vi "T3AWG Pick Rate.vi"(8 "error in (no error)":errorcluster, 10 "f0 [Hz]":dbl, 11 "t3awg":T1={"VISA"="", "use ext ref"=FALSE, "ext ref [Hz]"=0.0, "load Z"=enum."High Z", "ramdac max n"=0, "noise dither [V]"=0.0, "t3awg fs rules"=[], "channels"=0, "ramdac min n"=0, "channel list"=[], "gen resl [Vpp]"=0.0, "wave data format"=enum."Binary"} {"t3awg fs rules"."fs-step [Hz]" format="%#_6p"; "t3awg fs rules"."fs-max [Hz]" format="%#_6p"; "t3awg fs rules"."for f0 <" format="%#_6p"; "t3awg fs rules"."fs-min [Hz]" format="%#_6p"}) -> (0 "error out":errorcluster, 2 "fs-min [Hz]":dbl, 3 "t3awg out":T1={"VISA"="", "use ext ref"=FALSE, "ext ref [Hz]"=0.0, "load Z"=enum."High Z", "ramdac max n"=0, "noise dither [V]"=0.0, "t3awg fs rules"=[], "channels"=0, "ramdac min n"=0, "channel list"=[], "gen resl [Vpp]"=0.0, "wave data format"=enum."Binary"} {"t3awg fs rules"."fs-step [Hz]" format="%#_6p"; "t3awg fs rules"."fs-max [Hz]" format="%#_6p"; "t3awg fs rules"."for f0 <" format="%#_6p"; "t3awg fs rules"."fs-min [Hz]" format="%#_6p"})   [LabVIEW 2020, in "Active Technologies AWG3000.lvlib"]
uses:
  Active Technologies AWG3000.lvlib
  T3AWG Session.ctl
  T3AWG Load Z.ctl
  fgen_ramdac_fs_rules.ctl
  T3AWG Channel.ctl
  <vilib>/Utility/error.llb/Error Cluster From Error Code.vi
  <vilib>/ErrorRing/Error Ring.xnode
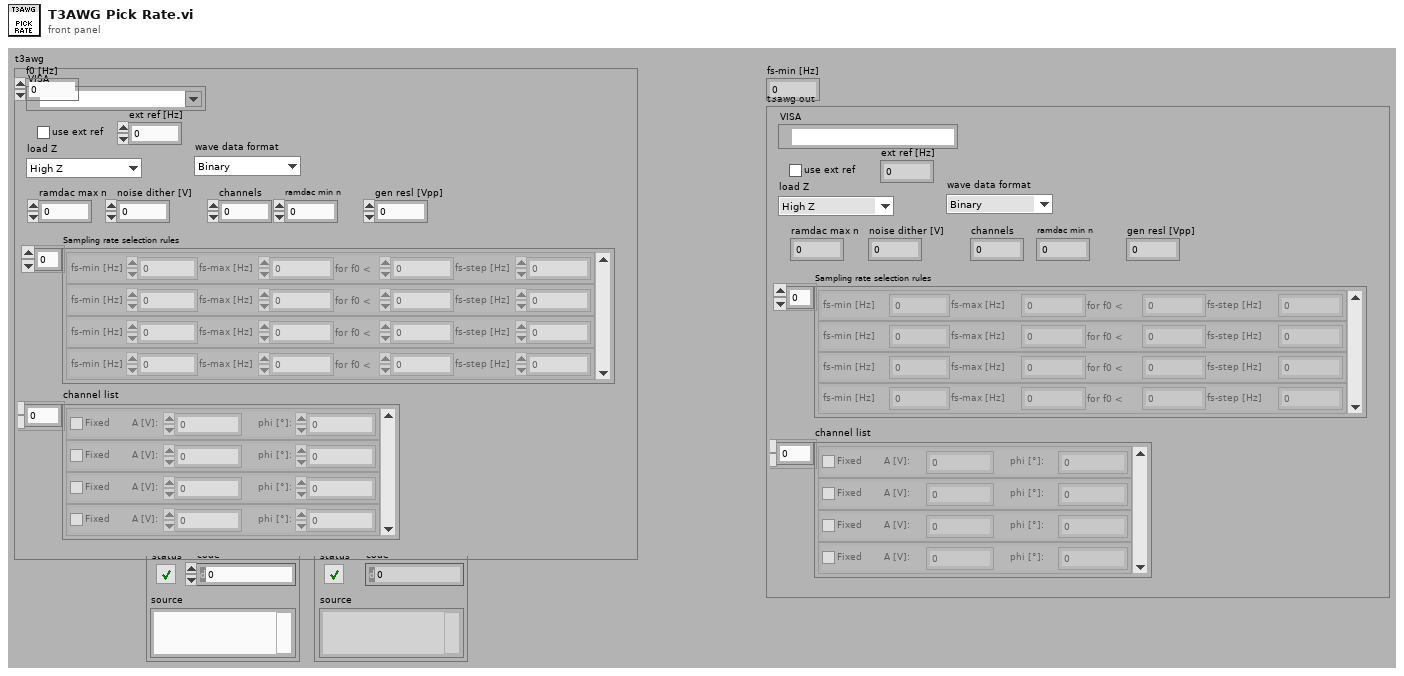
[diagram p1: front panel]
types:
  T1 = typedef "Active Technologies AWG3000.lvlib/T3AWG Session.ctl" = cluster{"VISA":refnum<visa-resource-name>, "use ext ref":bool, "ext ref [Hz]":dbl, "load Z":T2, "ramdac max n":i32, "noise dither [V]":dbl, "t3awg fs rules":T3[], "channels":i32, "ramdac min n":i32, "channel list":T4[], "gen resl [Vpp]":dbl, "wave data format":T5}
  T2 = typedef "Active Technologies AWG3000.lvlib/T3AWG Load Z.ctl" = enum16{"High Z", "50 Ohm"}
  T3 = typedef "Active Technologies AWG3000.lvlib/fgen_ramdac_fs_rules.ctl" = cluster{"fs-min [Hz]":dbl, "fs-max [Hz]":dbl, "for f0 < ":dbl, "fs-step [Hz]":dbl}
  T4 = typedef "Active Technologies AWG3000.lvlib/T3AWG Channel.ctl" = cluster{"Fixed":bool, "A [V]:":dbl, "phi [°]:":dbl}
  T5 = typedef "Active Technologies AWG3000.lvlib/T3AWG Wave Format" = enum16{"Text", "Binary"}
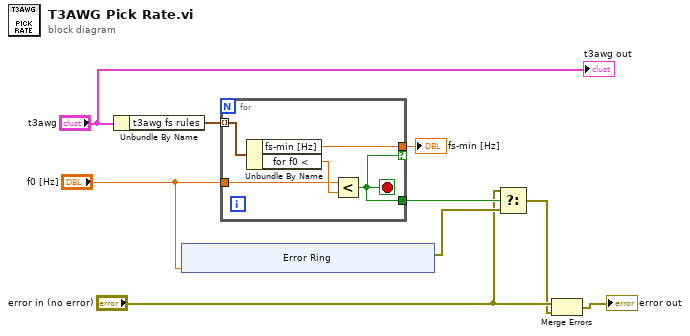
[diagram p0: block diagram]
diagram:
  n1 = Unbundle By Name("t3awg") -> ("t3awg fs rules"=w9:T3[])
  n2 = xnode "Error Ring"("parameter 0"="f0 [Hz]") -> ("error out"=w5:errorcluster)
  n3 = for {
    tunnel: w9 -> [w14] mode=indexing
    tunnel: "f0 [Hz]" -> [w12]
    tunnel: [w11] -> w8 if=w10
    tunnel: [w10] -> w6
    stop <- w10 stop-if-true
    n4 = Unbundle By Name(w14) -> ("fs-min [Hz]"=w11:dbl, "for f0 <"=w13:dbl)
    n5 = Less?(x=w12, y=w13) -> (x < y?=w10:bool)
  }
  "fs-min [Hz]" <- w8
  n6 = Select(t="error in (no error)", s=w6, f=w5) -> (s? t:f=w3:errorcluster)
  n7 = Merge Errors("error in (no error)", w3) -> (→"error out":errorcluster)
  "t3awg out" <- "t3awg"
